vi "B_d_load.vi"() -> ()   [LabVIEW 2022 SP3]
panel:
  out "size(s)":i32
  out "Init Data Out":sgl[](array[numeric])
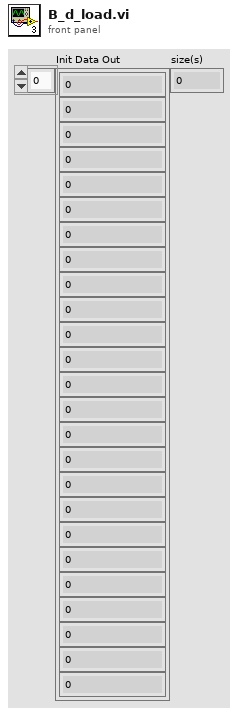
[diagram p1: front panel]
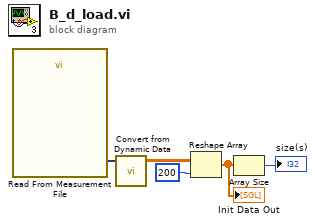
[diagram p0: block diagram]
diagram:
  n1 = call "Read From Measurement File"() -> ("Signals"=w4:dynamicdata)  [unwired: 6 in, 5 out]
  n2 = call "Convert from Dynamic Data"("Dynamic Data Type"=w4) -> ("Array"=w3:dbl[][])  [unwired: 3 in]
  n3 = Reshape Array(w3, 200 ("dimension size")) -> (w1:dbl[])
  "Init Data Out" <- w1
  n4 = Array Size(array=w1) -> (size(s)=→"size(s)":i32)
